vi "Create Symbol Information Loader.vi"(8 "error in (no error)":errorcluster, 11 "TwinCAT ADS in":refnum<class "TwinCAT ADS.lvclass">) -> (0 "error out":errorcluster, 1 "Symbol Info Loader":refnum<k24>, 3 "TwinCAT ADS out":refnum<class "TwinCAT ADS.lvclass">)   [LabVIEW 2018, in "TwinCAT ADS.lvclass"]
uses:
  TwinCAT ADS.lvclass
  TwinCAT.Ads
  TwinCAT ADS.lvclass/TwinCAT ADS.ctl
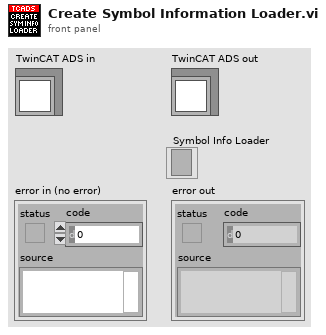
[diagram p1: front panel]
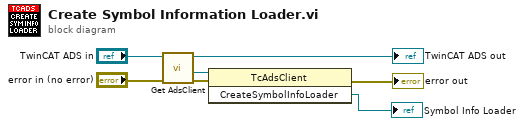
[diagram p0: block diagram]
diagram:
  n1 = call "Get AdsClient.vi"("error in (no error)"="error in (no error)", "TwinCAT ADS in"="TwinCAT ADS in") -> ("error out"=w2:errorcluster, ".NET TcAdsClient refnum"=w1:refnum<k24>, "TwinCAT ADS out"=→"TwinCAT ADS out":refnum<class "TwinCAT ADS.lvclass">)  [unwired: 7 in]
  n2 = invoke class="TcAdsClient" method="CreateSymbolInfoLoader"(reference=w1, error in=w2) -> (error out=→"error out":errorcluster, "CreateSymbolInfoLoader"=→"Symbol Info Loader":refnum<k24>)  [unwired: 1 in, 1 out]
